vi "ArraySum.vi"(11 "Array":i32[](array[numeric])) -> (3 "Sum":i32)   [LabVIEW 2013]
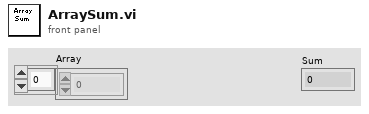
[diagram p1: front panel]
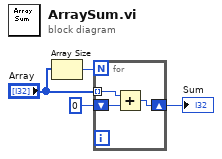
[diagram p0: block diagram]
diagram:
  n1 = Array Size(array="Array") -> (size(s)=w4:i32)
  n2 = for {
    N: w4 -> [_]
    shift-right: [w6] -> w2
    shift-left: 0 -> [w7]
    tunnel: "Array" -> [w5] mode=indexing
    n3 = Add(x=w5, y=w7) -> (x+y=w6:i32)
  }
  "Sum" <- w2
